vi "Database.Main.GetDBtime.vi"(8 "error in (no error)":errorcluster, 11 "Data in":T1 {"Variant"."TS"."TV"."minimum" format="%#.3f"; "Variant"."TS"."TV"."maximum" format="%#.3f"; "Variant"."TS"."TP"."value" format="%#.3f"}) -> (0 "error out":errorcluster, 3 "Data out":T1 {"Variant"."TS"."TV"."minimum" format="%#.3f"; "Variant"."TS"."TV"."maximum" format="%#.3f"; "Variant"."TS"."TP"."value" format="%#.3f"})   [LabVIEW 2016]
doc: "Get database time\n\nWabco 2017 All right reserved\nAuthor: maciej.szupienko@wabco-auto.com"
uses:
  Database.Main.Data.ctl
  Database.Main.Data.Status.ctl
  Database.Main.Data.Sets.ctl
  Database.Main.Data.Results.ctl
  ProdaNG/Controls/ProdaNG.Identification.ctl
  ProdaNG/Controls/ProdaNG.ProcessResult.ctl
  ProdaNG/Controls/ProdaNG.ProcessStepResult.ctl
  ProdaNG/Controls/ProdaNG.TestStepResult.ctl
  ProdaNG/Controls/ProdaNG.TestValueResult.ctl
  Database.Main.Data.Variant.ctl
  ProdaNG/Controls/ProdaNG.ProcessStepParam.ctl
  ProdaNG/Controls/ProdaNG.TestStep.ctl
  ProdaNG/Controls/ProdaNG.TestStepParam.ctl
  ProdaNG/Controls/ProdaNG.TestValue.ctl
  tools/EventLog/EventLog.EventSource.ctl
  <vilib>/Utility/miscctls.llb/LVDateTimeRec.ctl
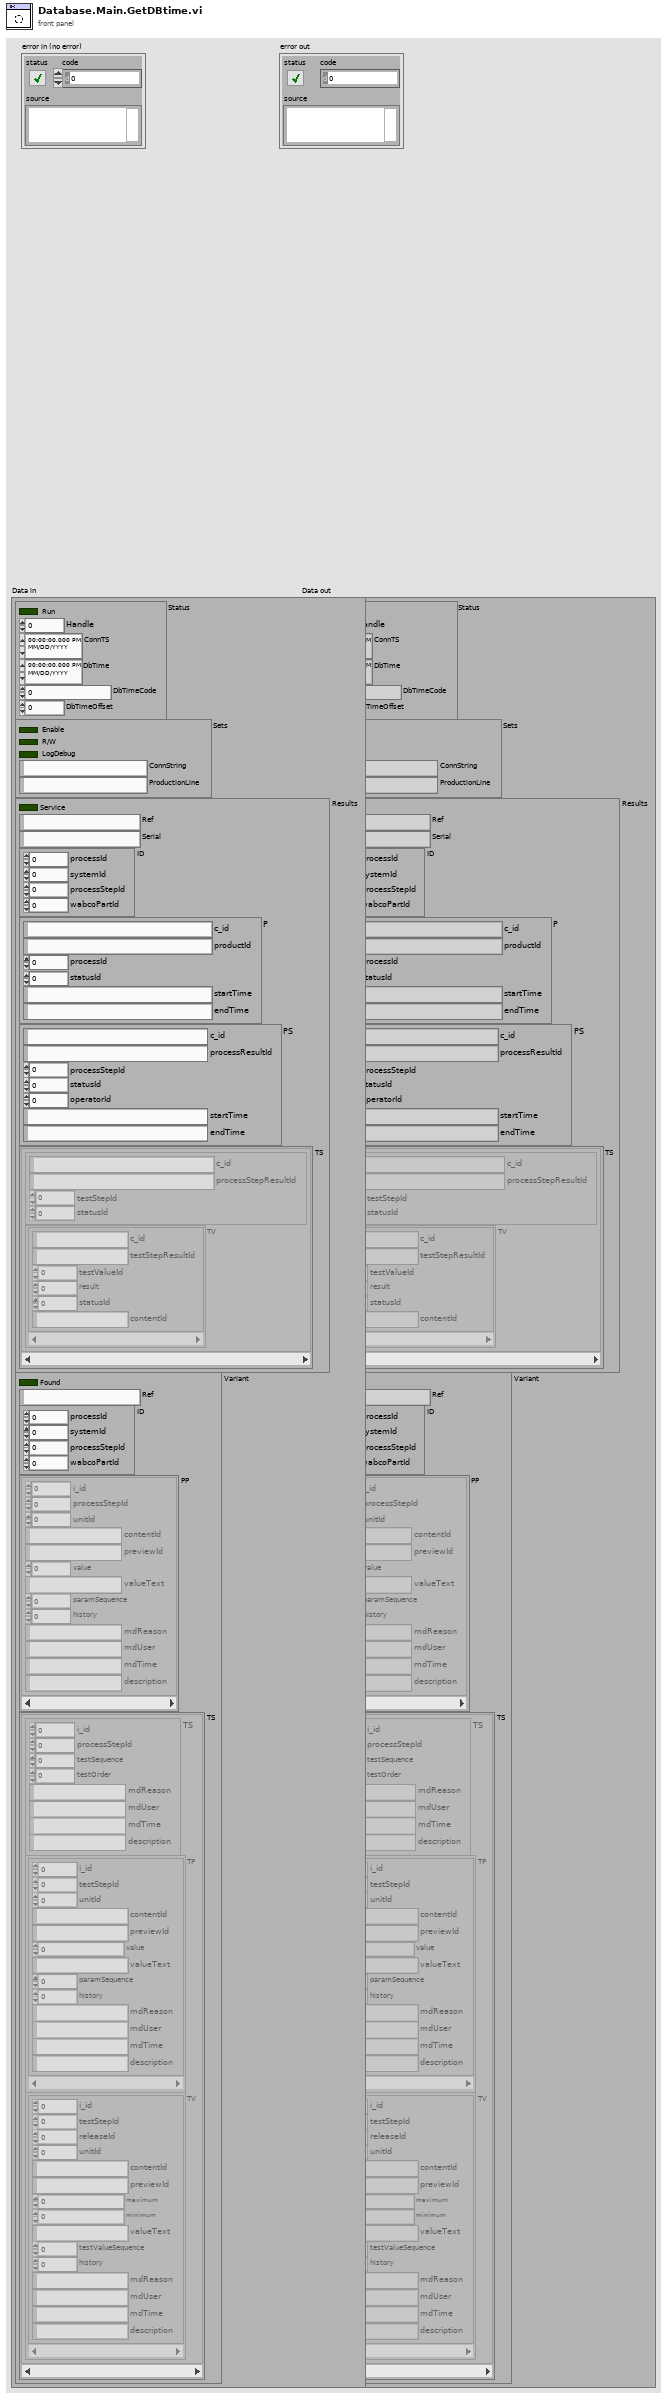
[diagram p1: front panel]
types:
  T1 = typedef "Database.Main.Data.ctl" = cluster{"Status":T2, "Sets":T3, "Results":T4, "Variant":T10}
  T2 = typedef "Database.Main.Data.Status.ctl" = cluster{"Run":bool, "Handle":i32, "ConnTS":timestamp, "DbTime":timestamp, "DbTimeCode":dbl, "DbTimeOffset":dbl}
  T3 = typedef "Database.Main.Data.Sets.ctl" = cluster{"Enable":bool, "R/W":bool, "LogDebug":bool, "ConnString":string, "ProductionLine":string}
  T4 = typedef "Database.Main.Data.Results.ctl" = cluster{"Service":bool, "Ref":string, "Serial":string, "ID":T5, "P":T6, "PS":T7, "TS":cluster{"TS":T8, "TV":T9[]}[]}
  T5 = typedef "ProdaNG.Identification.ctl" = cluster{"processId":i32, "systemId":i32, "processStepId":i32, "wabcoPartId":i32}
  T6 = typedef "ProdaNG.ProcessResult.ctl" = cluster{"c_id":string, "productId":string, "processId":i32, "statusId":i32, "startTime":string, "endTime":string}
  T7 = typedef "ProdaNG.ProcessStepResult.ctl" = cluster{"c_id":string, "processResultId":string, "processStepId":i32, "statusId":i32, "operatorId":i32, "startTime":string, "endTime":string}
  T8 = typedef "ProdaNG.TestStepResult.ctl" = cluster{"c_id":string, "processStepResultId":string, "testStepId":i32, "statusId":i32}
  T9 = typedef "ProdaNG.TestValueResult.ctl" = cluster{"c_id":string, "testStepResultId":string, "testValueId":i32, "result":dbl, "statusId":i32, "contentId":string}
  T10 = typedef "Database.Main.Data.Variant.ctl" = cluster{"Found":bool, "Ref":string, "ID":T5, "PP":T11[], "TS":cluster{"TS":T12, "TP":T13[], "TV":T14[]}[]}
  T11 = typedef "ProdaNG.ProcessStepParam.ctl" = cluster{"i_id":i32, "processStepId":i32, "unitId":i32, "contentId":string, "previewId":string, "value":dbl, "valueText":string, "paramSequence":i32, "history":i32, "mdReason":string, "mdUser":string, "mdTime":string, "description":string}
  T12 = typedef "ProdaNG.TestStep.ctl" = cluster{"i_id":i32, "processStepId":i32, "testSequence":i32, "testOrder":i32, "mdReason":string, "mdUser":string, "mdTime":string, "description":string}
  T13 = typedef "ProdaNG.TestStepParam.ctl" = cluster{"i_id":i32, "testStepId":i32, "unitId":i32, "contentId":string, "previewId":string, "value":dbl, "valueText":string, "paramSequence":i32, "history":i32, "mdReason":string, "mdUser":string, "mdTime":string, "description":string}
  T14 = typedef "ProdaNG.TestValue.ctl" = cluster{"i_id":i32, "testStepId":i32, "releaseId":i32, "unitId":i32, "contentId":string, "previewId":string, "maximum":dbl, "minimum":dbl, "valueText":string, "testValueSequence":i32, "history":i32, "mdReason":string, "mdUser":string, "mdTime":string, "description":string}
  T15 = typedef "EventLog.EventSource.ctl" = enum16{"All", "Gui", "Ref", "File", "Arch", "Seq", "CPX", "DB", "Laser", "Scan.P", "Scan.O"}
  T16 = typedef "LVDateTimeRec.ctl" = cluster{"fractional second":dbl, "second":i32, "minute":i32, "hour":i32, "day of month":i32, "month":i32, "year":i32, "day of week":i32, "day of year":i32, "DST":i32}
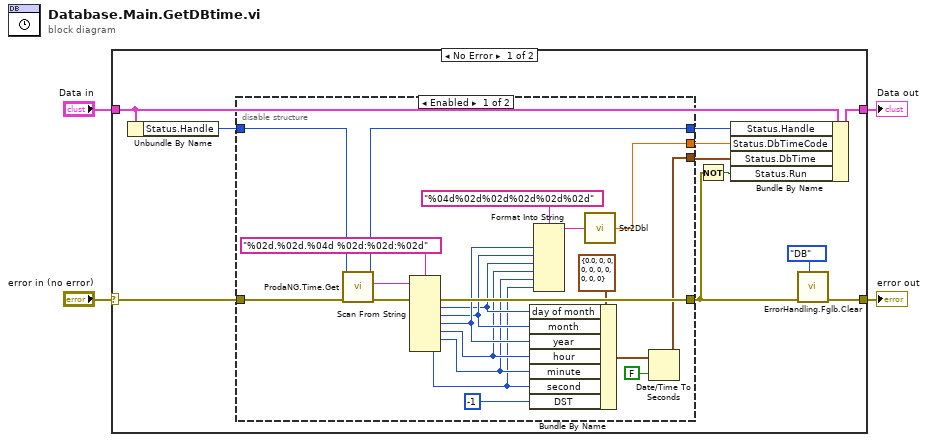
[diagram p0: block diagram]
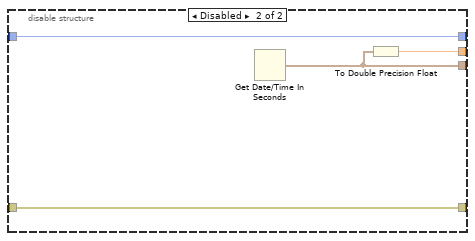
[diagram p2: hidden frame]
diagram:
  n1 = case shown="No Error" "error in (no error)" {
    selector: "error in (no error)" -> [w14 w42]
    tunnel: [w7 w42] -> w1
    tunnel: [w11 w41] -> w4
    tunnel: "Data in" -> [w12 w41]
    frame No Error {
      n2 = Unbundle By Name(w12) -> ("Status.Handle"=w13:i32)
      n3 = disable-structure shown="Enabled" {
        disable-tunnel: [w18 w37] -> w15
        disable-tunnel: w14 -> [w36 w40]
        disable-tunnel: w13 -> [w19 w37]
        disable-tunnel: [w16 w39] -> w10
        disable-tunnel: [w17 w38] -> w9
        disable-tunnel: [w35 w40] -> w5
        frame Enabled {
          n4 = call "ProdaNG.Time.Get.vi"("error in"=w36, "dbHandleIn"=w19) -> ("error out"=w33:errorcluster, "timeStr"=w21:string, "dbHandle"=w18:i32)  [unwired: 5 in, 1 out]
          n5 = Scan From String(format string="%02d.%02d.%04d %02d:%02d:%02d", input string=w21, error in=w33) -> (error out=w35:errorcluster, output 1=w26:i32, output 2=w27:i32, output 3=w28:i32, output 4=w25:i32, output 5=w24:i32, output 6=w23:i32)  [unwired: 7 in, 2 out]
          n6 = Bundle By Name(cluster=T16 {"fractional second"=0.0, "second"=0, "minute"=0, "hour"=0, "day of month"=0, "month"=0, "year"=0, "day of week"=0, "day of year"=0, "DST"=0} ("date time rec"), "day of month"=w26, "month"=w27, "year"=w28, "hour"=w25, "minute"=w24, "second"=w23, "DST"=-1) -> (w31:T16)
          n7 = Format Into String(format string="%04d%02d%02d%02d%02d%02d", w28, w27, w26, w25, w24, w23) -> (resulting string=w20:string)  [unwired: 2 in, 1 out]
          n8 = call "Str2Dbl.vi"("string"=w20) -> ("Numeric"=w17:dbl)
          n9 = Date/Time To Seconds(1:FALSE ("is UTC (F)"), 2:w31) -> (0:w16:timestamp)
        }
        frame Disabled {
          n10 = Get Date/Time In Seconds() -> (seconds since 1Jan1904=w39:timestamp)
          n11 = To Double Precision Float(number=w39) -> (double precision float=w38:dbl)
        }
      }
      n12 = Not(x=w5) -> (.not. x?=w6:bool)
      n13 = Bundle By Name(cluster=w12, "Status.Handle"=w15, "Status.DbTimeCode"=w9, "Status.DbTime"=w10, "Status.Run"=w6) -> (w11:T1)
      n14 = call "ErrorHandling.Fglb.Clear.vi"("Event source"=EventLog.EventSource."DB", "error in (no error)"=w5) -> ("error out"=w7:errorcluster)  [unwired: 9 in]
    }
    frame Error {
    }
  }
  "error out" <- w1
  "Data out" <- w4
